vi "Window-Ini file load error message.vi"(6 "Mention app will exit? (F)":bool, 8 "error in (no error)":errorcluster, 11 "Message":string) -> (0 "Error Out (no error)":errorcluster)   [LabVIEW 2013]
uses:
  <vilib>/Utility/error.llb/DialogType.ctl
  Global Variables/General Globals.vi
panel:
  out "error out":errorcluster
  in  "Close":bool
  out "Message":string
  in  "Vertical Stop Button":bool
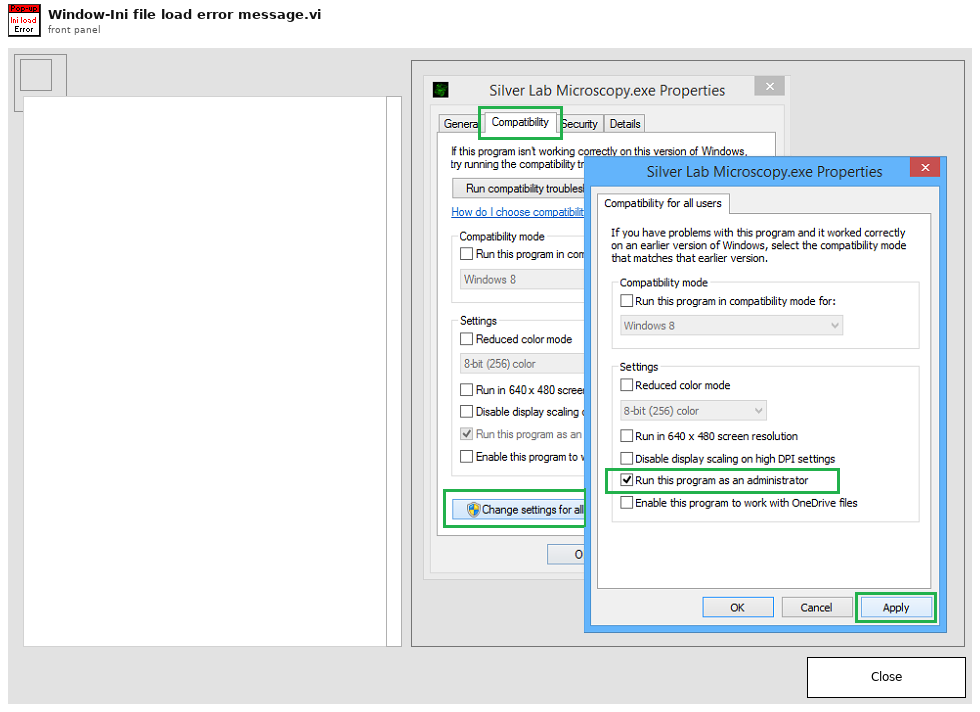
[diagram p1: front panel]
types:
  T1 = enum32{"invalid app kind", "Development System", "Run Time System", "Student Edition", "Embedded LabVIEW", "Evaluation", "Custom"}
  T2 = typedef "DialogType.ctl" = u16
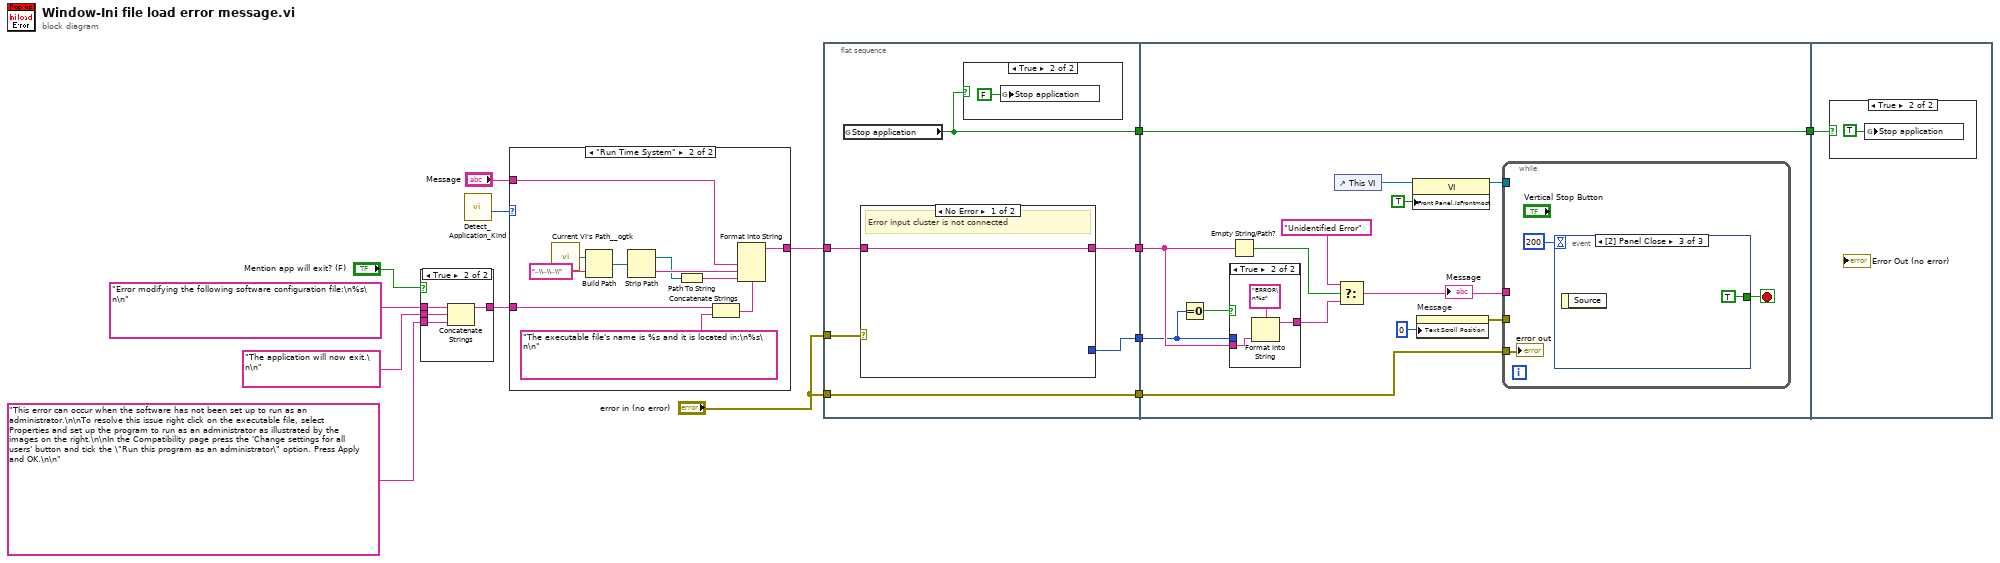
[diagram p0: block diagram]
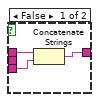
[diagram p2: hidden frame]
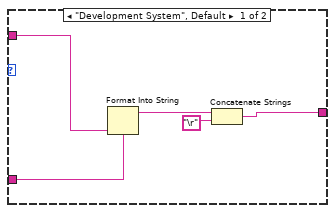
[diagram p3: hidden frame]
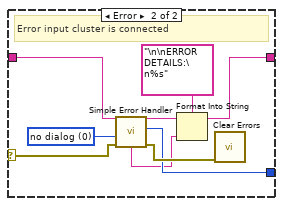
[diagram p4: hidden frame]
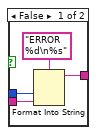
[diagram p6: hidden frame]
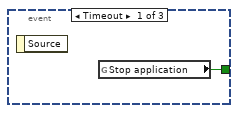
[diagram p7: hidden frame]
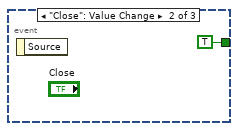
[diagram p8: hidden frame]
diagram:
  n1 = case shown="True" "Mention app will exit? (F)" {
    tunnel: "Error modifying the following software configuration file:\n%s\n\n" ("message") -> [w16 w21]
    tunnel: [w15 w19] -> w7
    tunnel: "The application will now exit.\n\n" ("message") -> [_ w20]
    tunnel: "This error can occur when the software has not been set up to run as an administrator.\n\nTo resolve this issue right click on the executable file, select Properties and set up the program to run as an administrator as illustrated by the images on the right.\n\nIn the Compatibility page press the 'Change settings for all users' button and tick the \"Run this program as an administrator\" option. Press Apply and OK.\n\n" ("message") -> [w17 w18]
    frame False {
      n2 = Concatenate Strings(w16, w17) -> (w15:string)
    }
    frame True {
      n3 = Concatenate Strings(w21, w20, w18) -> (w19:string)
    }
  }
  n4 = call "Detect_Application_Kind.vi"() -> ("Application:Kind"=w1:T1)  [unwired: 9 in, 2 out]
  n5 = case shown="\"Run Time System\"" w1 {
    tunnel: w7 -> [w25 w34]
    tunnel: "Message" -> [w26 w35]
    tunnel: [w23 w28] -> w9
    frame "Development System", Default {
      n6 = Format Into String(format string=w25, w26) -> (resulting string=w24:string)  [unwired: 2 in, 1 out]
      n7 = Concatenate Strings(w24, "\r") -> (w23:string)
    }
    frame "Run Time System" {
      n8 = call "Current VI's Path__ogtk.vi"() -> ("Current VI's Path (+ Relative)"=w36:path)  [unwired: 1 in]
      n9 = Build Path(base path=w36, name or relative path="..\\..\\..\\") -> (appended path=w32:path)
      n10 = Strip Path(path=w32) -> (stripped path=w27:path, name=w31:string)
      n11 = Path To String(path=w27) -> (string=w30:string)
      n12 = Concatenate Strings(w34, "The executable file's name is %s and it is located in:\n%s\n\n" ("message")) -> (w33:string)
      n13 = Format Into String(format string=w33, w35, w31, w30) -> (resulting string=w28:string)  [unwired: 2 in, 1 out]
    }
  }
  n14 = flat-sequence {
    tunnel: [w41] -> w14
    tunnel: [w40] -> w12
    tunnel: w9 -> [w42]
    tunnel: "error in (no error)" -> [w43]
    tunnel: [w39] -> w11
    tunnel: "error in (no error)" -> [w38]
    tunnel: [w38] -> w3
    tunnel: w14 -> [w57]
    tunnel: [w61] -> w13
    tunnel: w12 -> [w61]
    tunnel: w11 -> [w55]
    tunnel: w3 -> [w54]
    tunnel: w13 -> [w81]
    frame #0 {
      n15 = global read "General Globals.vi" "Stop application"() -> (w40:bool)
      n16 = case shown="No Error" w43 {
        selector: w43 -> [_ w48]
        tunnel: w42 -> [w44 w46]
        tunnel: [w44 w49] -> w41
        tunnel: [_ w47] -> w39
        frame No Error {
          # "Error input cluster is not connected"
        }
        frame Error {
          w52 = T2 0 items=["no dialog", "OK message", "continue or stop message", "OK message + warnings", "continue/stop + warnings"] ("type of dialog (OK msg:1)")
          # "Error input cluster is connected"
          n17 = call <vilib>:"Simple Error Handler.vi"("type of dialog (OK msg:1)"=w52, "error in (no error)"=w48) -> ("code out"=w47:i32, "error out"=w50:errorcluster, "message"=w45:string)  [unwired: 3 in, 2 out]
          n18 = Format Into String(format string="\n\nERROR DETAILS:\n%s", initial string=w46, w45) -> (resulting string=w49:string)  [unwired: 1 in, 1 out]
          n19 = call <vilib>:"Clear Errors.vi"("error in (no error)"=w50) -> ()  [unwired: 6 in, 1 out]
        }
      }
      n20 = case shown="True" w40 {
        frame False {
        }
        frame True {
          n21 = global write "General Globals.vi" "Stop application"(FALSE ("Quit?")) -> ()
        }
      }
    }
    frame #1 {
      n22 = Equal To 0?(x=w55) -> (x = 0?=w56:bool)
      n23 = case shown="True" w56 {
        tunnel: [w71 w74] -> w62
        tunnel: w57 -> [w70 w72]
        tunnel: w55 -> [w69 _]
        frame False {
          n24 = Format Into String(format string="ERROR %d\n%s", w69, w70) -> (resulting string=w71:string)  [unwired: 2 in, 1 out]
        }
        frame True {
          n25 = Format Into String(format string="ERROR\n%s", w72) -> (resulting string=w74:string)  [unwired: 2 in, 1 out]
        }
      }
      n26 = Empty String/Path?(string/path=w57) -> (empty?=w67:bool)
      n27 = control-ref of="This VI"() -> (w59:refnum<vi>)
      n28 = Select(t="Unidentified Error" ("String"), s=w67, f=w62) -> (s? t:f=w63:string)
      "Message" <- w63
      n29 = property on="Property Node" class="VI"(reference=w59, "Front Panel.IsFrontmost"=TRUE ("Front Panel Window:Is Frontmost")) -> (reference out=w58:refnum<vi>)  [unwired: 1 in, 1 out]
      n30 = property on="Message" class="Str"("Text.Scroll Position"=u32 0) -> (error out=w64:errorcluster)  [unwired: 2 in, 1 out]
      n31 = while {
        tunnel: w63 -> [_]
        tunnel: w64 -> [_]
        tunnel: w58 -> [_]
        tunnel: w54 -> [w75]
        stop <- w77 stop-if-true
        n32 = event shown="[2] Panel Close" {
          selector: _ -> [_ _ _]
          dyn-events: _ -> [_ _ _]
          timeout: 200 -> [_ _ _]
          tunnel: [w78 TRUE ("Stop?") TRUE ("Stop?")] -> w77
          event Timeout {
            n33 = event-data() -> ()  [unwired: 1 in, 1 out]
            n34 = global read "General Globals.vi" "Stop application"() -> (w78:bool)
          }
          event "Close": Value Change {
            n35 = event-data() -> ()  [unwired: 1 in, 1 out]
          }
          event Panel Close {
            n36 = event-data() -> ()  [unwired: 1 in, 1 out]
          }
        }
        "error out" <- w75
      }
    }
    frame #2 {
      n37 = case shown="True" w81 {
        frame False {
        }
        frame True {
          n38 = global write "General Globals.vi" "Stop application"(TRUE ("Quit?")) -> ()
        }
      }
    }
  }
